vi "CLSUIP_ShouldReplaceControl.vi"(4 "error in (no error)":errorcluster, 5 "Terminal Index":u32, 6 "ConPane":refnum<vi>, 7 "VIRetooler":refnum<class "OverrideRetooler.lvclass">) -> (0 "error out":errorcluster, 1 "Should replace?":bool, 3 "VIRetooler 2":refnum<class "OverrideRetooler.lvclass">)   [LabVIEW 2021, in "MemberVICreation.lvlib" / "OverrideRetooler.lvclass"]
uses:
  <resource>/Framework/Providers/LVClassLibrary/NewAccessors/OverrideRetooler/OverrideRetooler.lvclass
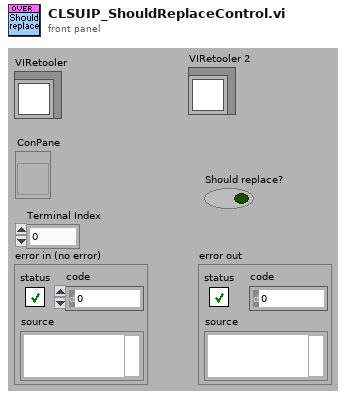
[diagram p1: front panel]
types:
  T1 = enum16{"Invalid Wire Rule", "Required", "Recommended", "Optional", "Dynamic Dispatch"}
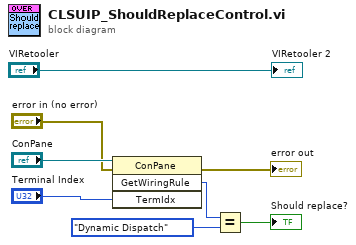
[diagram p0: block diagram]
diagram:
  n1 = invoke class="ConPane" method="GetWiringRule"(reference="ConPane", error in="error in (no error)", "TermIdx"="Terminal Index") -> (error out=→"error out":errorcluster, "Get Wire Rule"=w6:T1)  [unwired: 1 in, 2 out]
  n2 = Equal?(x=w6, y=T1."Dynamic Dispatch") -> (x = y?=→"Should replace?":bool)
  "VIRetooler 2" <- "VIRetooler"
